vi "Build.vi"(8 "error in (no error)":errorcluster, 11 "Build in":refnum<class "AB_PackedLibrary.lvclass">) -> (0 "error out":errorcluster, 1 "GeneratedFiles":path[](array[path]), 2 "GeneratedDirectories":path[](array[path]), 3 "Build out":refnum<class "AB_PackedLibrary.lvclass">, 4 "GeneratedFileGUIDs":string[](array[string]), 5 "OutputDirectory":path, 7 "Dependencies":T1[](array[typedef]))   [LabVIEW 2020, in "AB_PackedLibrary.lvclass"]
uses:
  <vilib>/AppBuilder/AB_Classes/PackedLib/AB_PackedLibrary.lvclass
  e:/builds/penguin/labview/branches/2020/dev/dist/vi.lib/AppBuilder/AB_Classes/Build/AB_Build.lvclass
  e:/builds/penguin/labview/branches/2020/dev/dist/vi.lib/AppBuilder/AB_Classes/TargetFile/AB_Targetfile.lvclass
  <vilib>/AppBuilder/AB_Dependency.ctl
  <vilib>/Utility/lvfile.llb/LVFileType.ctl
  <vilib>/AppBuilder/AB_Classes/PackedLib/AB_PackedLibrary.lvclass/AB_PackedLibrary.ctl
  <resource>/Framework/Providers/Common/provcom_StringGlobals.vi
  <vilib>/AppBuilder/AB_Classes/Source/AB_Source.lvclass
  <vilib>/AppBuilder/AB_Classes/TargetFile/AB_Targetfile.lvclass
  <vilib>/AppBuilder/AB_Classes/Destination/AB_Destination.lvclass
  <vilib>/AppBuilder/AB_Classes/Build/AB_Build.lvclass
  <vilib>/Utility/lvfile.llb/NI_FileType.lvlib
panel:
  out "error out 2":errorcluster
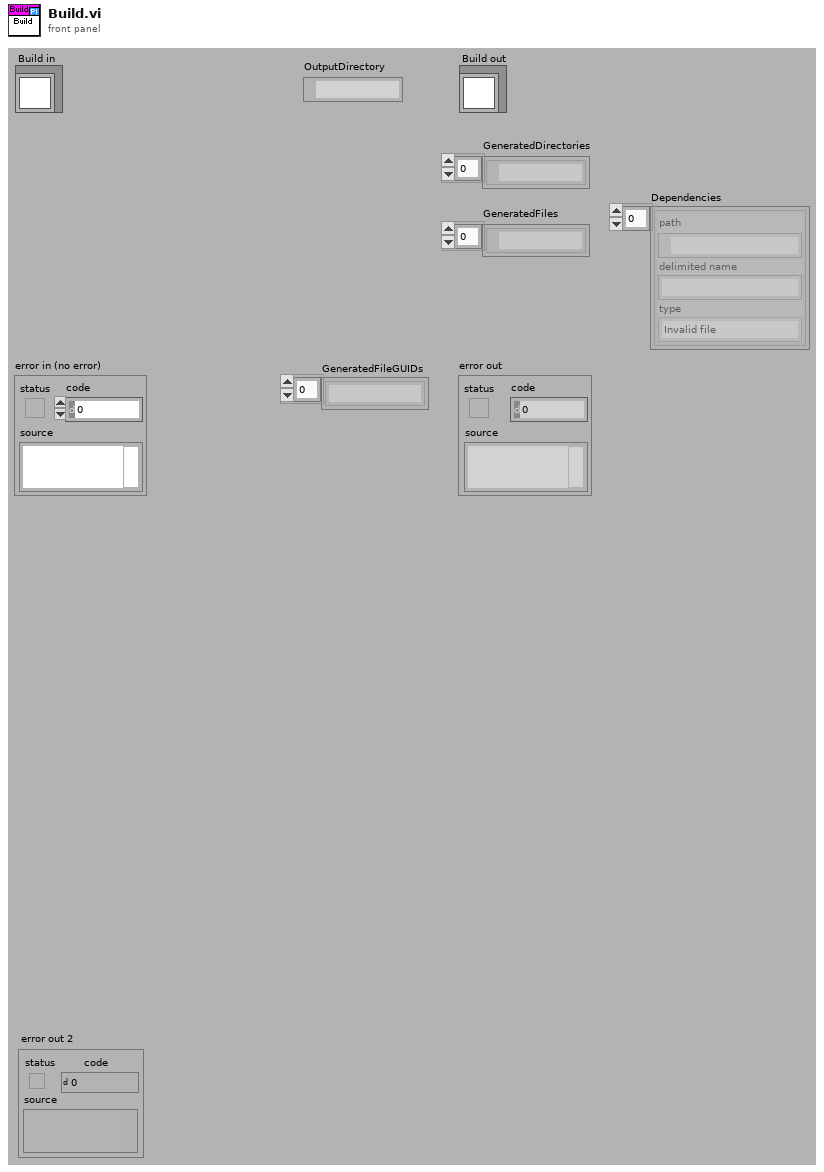
[diagram p1: front panel]
types:
  T1 = typedef "AB_Dependency.ctl" = cluster{"path":path, "delimited name":string, "type":T2}
  T2 = typedef "NI_FileType.lvlib/LVFileType.ctl" = enum32{"Invalid file", "Unknown type", "Instrument", "Control", "Polymorphic VI", "Project", "Library", "LVClass", "XControl", "XNode", "Shared library", ".NET assembly", "ActiveX interface", "CIN", "Run-time menu", "Palette menu", "Help file", "LLB", "XNode Edit Dependency", "Class Private Data Control", "Statechart", "MathScript .m file", "Ladder Diagram", "LVLibp", "XNode Build Dependency"}
  T3 = typedef "AB_Source.ctl" = cluster{"path":path, "itemID":string, "parentIndex":i32, "sourceInclusion":T4, "destinationIndex":i32, "properties":T5[], "newName":string, "lvfile":bool, "valid":bool, "eng_inBuild":bool, "eng_isNonVILink":bool, "Amalgamation":bool, "Amalgamation Piece":bool, "eng_delimitedName":string, "preventRename":bool}
  T4 = typedef "AB_Source_Inclusion.ctl" = enum16{"IncludeIfReferenced", "Include", "Exclude", "TopLevel"}
  T5 = typedef "AB_Source_Properties.ctl" = cluster{"sourcePropertyType":T6, "value":variant}
  T6 = typedef "AB_Source_Property_Type.ctl" = enum16{"Remove block diagram", "Remove front panel", "Password", "Window has title bar", "Show menu bar", "Show vertical scroll bar", "Show horizontal scroll bar", "Show toolbar", "Show Abort button", "Show fp when called", "Window behavior", "Allow user to close window", "Window run-time position", "Run when opened", "Allow debugging", "Auto error handling", "Generate guard code", "Use stack variables", "Expression folding", "Integer only", "Inline subVI"}
  T7 = typedef "AB_Build.ctl" = cluster{"buildSpecName":string, "buildSpecDescription":string, "destinations":refnum<class "AB_Destination.lvclass">[], "exclusionOption":T8, "defaultLanguage":string, "supportedLanguages":string[], "excludedDirectories":path[], "buildContext":refnum<vi>, "buildObject":T9, "preview":bool, "programatic":bool, "progressBarEvents":T10, "userLog_Path":path, "preActionID":string, "preAction_Path":path, "postActionID":string, "postAction_Path":path, "eng_checkForBrokenVIs?":bool, "eng_verboseLinkerErrors?":bool, "localDest_Path":path, "targetDest_Path":path, "removeVIObject":u16, "cache":refnum<class "PreviewCache.lvclass">, "use cache":bool, "previewCache_ID":string, "buildCache_ID":string, "eng_TempLocalDest_Path":path, "eng_collectDependencies?":bool, "versionInfo":cluster{"buildVersion":cluster{"major":u16, "minor":u16, "patch":u16, "build":u16}, "autoIncrement":bool}, "eng_enableVIChecksums":bool}
  T8 = typedef "AB_Exclusion_Option.ctl" = cluster{"typedefs":bool, "polymorphicVIs":bool, "unusedLibraryItems":bool, "modifyLibraryFile":bool, "edit-timeDependencies":bool, "inlineVIs":bool, "dependent PPLs":bool, "dependent DLLs":bool}
  T9 = typedef "ItemRef.ctl" = u64
  T10 = typedef "provcom_ProgressBar_Events.ctl" = cluster{"newJob":refnum<user-event>, "newItem":refnum<user-event>, "errorMsg":T11, "cancel":refnum<user-event>}
  T11 = typedef "mxLvBuildError.ctl" = refnum<user-event>
  T12 = typedef "AB_Targetfile.ctl" = cluster{"targetfileName":string, "targetfileGUID":string, "enableDebugging":bool, "versionInfo":cluster{"productName":string, "legalCopyright":string, "companyName":string, "internalName":string, "fileDescription":string}, "eng_consolidatedTypeInfo":string, "fastFileFormat":bool, "eng_LEIFBuildData":u32, "versionIndependent":bool}
  T13 = typedef "AB_CopyFiles_Data.ctl" = cluster{"processedItems":T14[]}
  T14 = typedef "AB_Source_Processed_Info.ctl" = cluster{"destPath":path, "buildDelimitedName":string, "sourceIndex":i32, "topLevel":bool}
  T15 = typedef "AB_Destination.ctl" = cluster{"destName":string, "path":path, "libraryName":string, "preserveHierarchy":bool, "eng_inBuild":bool, "eng_libraryReference":refnum<vi>, "eng_restictAddToNewLibrary":bool}
  T16 = typedef "AB_Version_Info.ctl" = cluster{"PrivateBuild":string, "SpecialBuild":string, "LegalCopyright":string, "LegalTrademarks":string, "Comments":string, "FileDescription":string, "InternalName":string, "file version":cluster{"major":u16, "minor":u16, "patch":u16, "build":u16}, "ProductName":string, "FileType":u16, "CompanyName":string, "OriginalFilename":string}
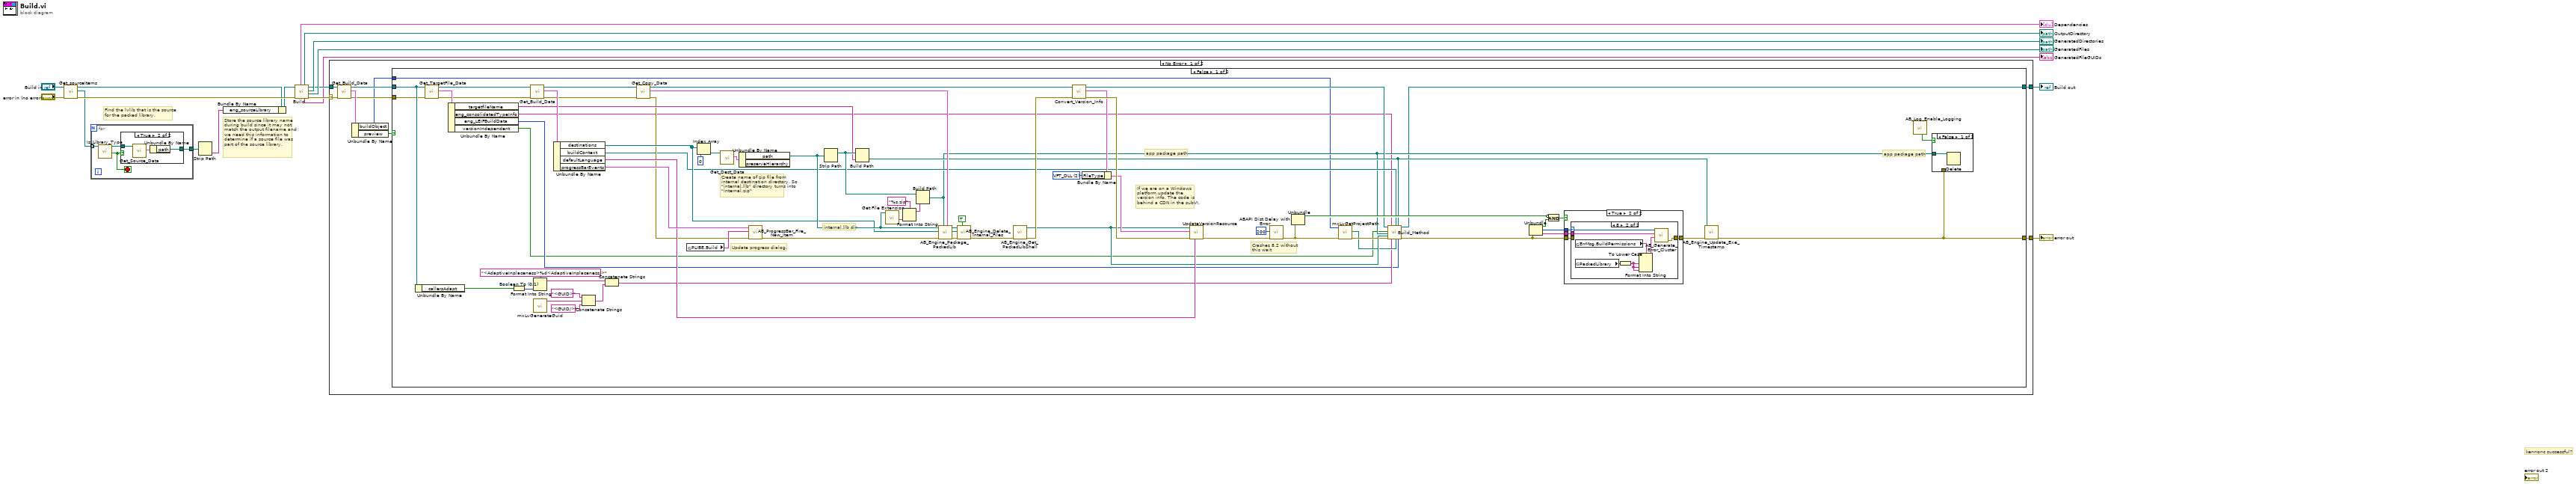
[diagram p0: block diagram]
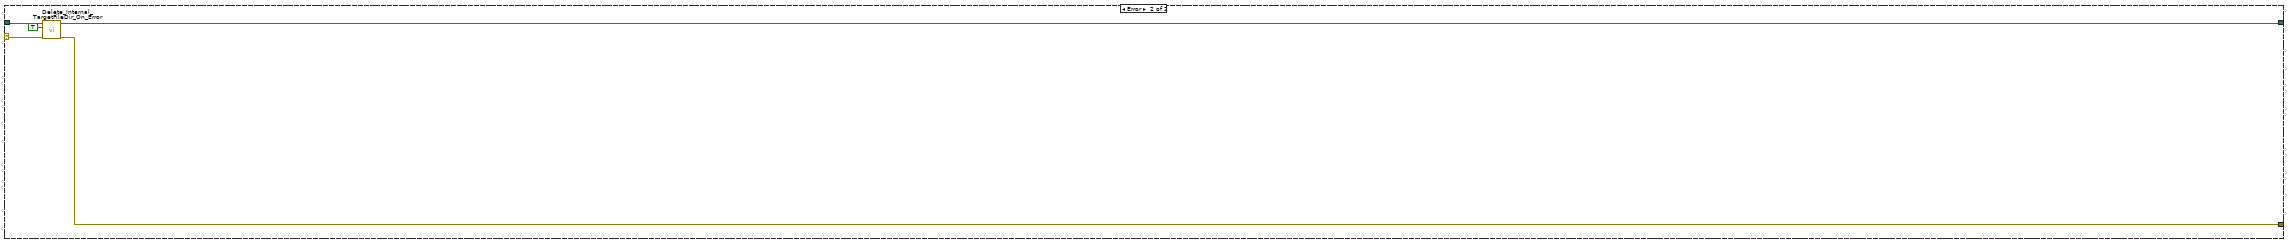
[diagram p7: hidden frame]
diagram:
  # "Store the source library name during build since it may not match the output filename and we need this information to determine if a source file was part of the source library."
  # "Find the lvlib that is the source for the packed library."
  # "kennonc successful?"
  n1 = call <vilib>:"Get_sourceItems.vi"("error in (no error)"="error in (no error)", "Class in"="Build in") -> ("error out"=w7:errorcluster, "sourceItems"=w6:refnum<class "AB_Source.lvclass">[], "Class out"=w4:refnum<class "AB_PackedLibrary.lvclass">)  [unwired: 7 in]
  n2 = for {
    tunnel: w6 -> [w21] mode=indexing
    tunnel: [w19] -> w5
    stop <- w18 stop-if-true
    n3 = call-dynamic "Is_Library_Type.vi"("AB_Source in"=w21) -> ("LVLIBPtopLevel"=w18:bool, "AB_Source out"=w20:refnum<class "AB_Source.lvclass">)  [unwired: 1 in, 8 out]
    n4 = case shown="True" w18 {
      tunnel: w20 -> [_ w22]
      tunnel: [_ w24] -> w19
      frame False {
      }
      frame True {
        n5 = call <vilib>:"Get_Source_Data.vi"("Class in"=w22) -> ("data"=w23:T3)  [unwired: 1 in, 9 out]
        n6 = Unbundle By Name(w23) -> ("path"=w24:path)
      }
    }
  }
  n7 = Strip Path(path=w5) -> (name=w2:string)  [unwired: 1 out]
  n8 = Bundle By Name(cluster=w4, "eng_sourceLibrary"=w2) -> (w3:refnum<class "AB_PackedLibrary.lvclass">)
  n9 = call-parent "Build.vi"("error in (no error)"=w7, "Build in"=w3) -> ("error out"=w12:errorcluster, "GeneratedFiles"=→"GeneratedFiles":path[], "GeneratedDirectories"=→"GeneratedDirectories":path[], "Build out"=w13:refnum<class "AB_PackedLibrary.lvclass">, "GeneratedFileGUIDs"=→"GeneratedFileGUIDs":string[], "OutputDirectory"=→"OutputDirectory":path, "Dependencies"=→"Dependencies":T1[])  [unwired: 3 out]
  n10 = case shown="No Error" w12 {
    selector: w12 -> [w27 w121]
    tunnel: [w33 w119] -> w15
    tunnel: [w32 w120] -> w14
    tunnel: w13 -> [w31 w122]
    frame No Error {
      n11 = call <vilib>:"Get_Build_Data.vi"("error in (no error)"=w27, "Class in"=w31) -> ("error out"=w26:errorcluster, "data"=w30:T7, "Class out"=w28:refnum<class "AB_PackedLibrary.lvclass">)  [unwired: 7 out]
      n12 = Unbundle By Name(w30) -> ("buildObject"=w25:T9, "preview"=w29:bool)
      n13 = case shown="False" w29 {
        tunnel: [w37 w117] -> w33
        tunnel: [w38 w116] -> w32
        tunnel: w28 -> [w83 w117]
        tunnel: w26 -> [w82 w116]
        tunnel: w25 -> [w46 _]
        frame False {
          w97 = u16 2 items=["VFT_UNKNOWN", "VFT_APP", "VFT_DLL", "VFT_DRV", "VFT_FONT", "VFT_VXD", "-", "VFT_STATIC_LIB"] ("FileType")
          # "app package path"
          # "Crashes 8.2 without\nthis wait"
          # "Create name of zip file from internal destination directory. So \"internal.llb\" directory turns into \"internal.zip\""
          # "internal.llb dir"
          # "app package path"
          # "Update progress dialog."
          # "If we are on a Windows platform,update the version info. The code is behind a CDN in the subVI."
          n14 = Unbundle By Name(w83) -> ("callersAdapt"=w57:bool)
          n15 = call <vilib>:"Get_TargetFile_Data.vi"("error in (no error)"=w82, "AB_Targetfile in"=w83) -> ("error out"=w81:errorcluster, "data"=w84:T12, "AB_Targetfile out"=w79:refnum<class "AB_PackedLibrary.lvclass">)  [unwired: 7 in]
          n16 = Unbundle By Name(w84) -> ("targetfileName"=w80:string, "eng_consolidatedTypeInfo"=w49:string, "eng_LEIFBuildData"=w35:u32, "versionIndependent"=w34:bool)
          n17 = Boolean To (0,1)(Boolean=w57) -> (0, 1=w56:i16)
          n18 = call <vilib>:"Get_Build_Data.vi"("error in (no error)"=w81, "Class in"=w79) -> ("error out"=w62:errorcluster, "data"=w99:T7, "Class out"=w64:refnum<class "AB_PackedLibrary.lvclass">)  [unwired: 7 out]
          n19 = Format Into String(format string="<AdaptiveInplaceness>%d<AdaptiveInplaceness/>", w56) -> (resulting string=w44:string)  [unwired: 2 in, 1 out]
          n20 = call <resource>:"mxLvGenerateGuid.vi"() -> ("Value"=w42:string)  [unwired: 10 in, 1 out]
          n21 = Unbundle By Name(w99) -> ("destinations"=w85:refnum<class "AB_Destination.lvclass">[], "buildContext"=w54:refnum<vi>, "defaultLanguage"=w86:string, "progressBarEvents"=w94:T10)
          n22 = Concatenate Strings("<GUID>" ("string"), w42, "<GUID/>" ("string")) -> (w39:string)
          n23 = Concatenate Strings(w44, w39) -> (w43:string)
          n24 = call <vilib>:"Get_Copy_Data.vi"("error in (no error)"=w62, "AB_Build in"=w64) -> ("error out"=w61:errorcluster, "copyData"=w60:T13, "AB_Build out"=w63:refnum<class "AB_PackedLibrary.lvclass">)  [unwired: 7 in]
          n25 = global read "provcom_StringGlobals.vi" "PLIBE.Build"() -> (w95:string)
          n26 = Index Array(array=w85, index=0) -> (element=w89:refnum<class "AB_Destination.lvclass">)
          n27 = call <vilib>:"Get_Dest_Data.vi"("Class in"=w89) -> ("destName"=w100:T15)  [unwired: 1 in, 9 out]
          n28 = Unbundle By Name(w100) -> ("path"=w88:path)  [unwired: 1 out]
          n29 = call <vilib>:"AB_ProgressBar_Fire_New_Item.vi"("error in (no error)"=w61, "Label"=w95, "progressBarEvents in"=w94) -> ("error out"=w92:errorcluster)  [unwired: 8 out]
          n30 = Strip Path(path=w88) -> (stripped path=w90:path)  [unwired: 1 out]
          n31 = Build Path(base path=w90, name or relative path=w80) -> (appended path=w55:path)
          n32 = call <vilib>:"Get File Extension.vi"("file"=w88) -> ("filename without extension"=w70:string)  [unwired: 1 in, 9 out]
          n33 = Format Into String(format string="%s.zip", w70) -> (resulting string=w69:string)  [unwired: 2 in, 1 out]
          n34 = Build Path(base path=w90, name or relative path=w69) -> (appended path=w52:path)
          n35 = call <vilib>:"AB_Engine_Package_PackedLib.vi"("processed_sourceItems"=w60, "application package path"=w52, "error in (no error)"=w92, "destinations"=w85, "internal directory"=w88) -> ("error out"=w67:errorcluster, "support dir"=w65:path, "dup internal directory"=w66:path)  [unwired: 4 in]
          n36 = call <vilib>:"AB_Engine_Delete_Internal_Files.vi"("override Mac support directory preservation"=TRUE ("is Packed Library?"), "error in (no error)"=w67, "support dir"=w65, "internal directory"=w66) -> ("error out"=w91:errorcluster)  [unwired: 7 in]
          n37 = call <vilib>:"AB_Engine_Get_PackedLibShell.vi"("error in (no error)"=w91) -> ("error out"=w78:errorcluster, "pathPackedLibShell"=w51:path)  [unwired: 9 in]
          n38 = call-dynamic "Convert_Version_Info.vi"("error in (no error)"=w78, "AB_Targetfile in"=w63) -> ("error out"=w98:errorcluster, "input version info"=w96:T16, "AB_Targetfile out"=w53:refnum<class "AB_PackedLibrary.lvclass">)  [unwired: 7 out]
          n39 = Bundle By Name(cluster=w96, "FileType"=w97) -> (w93:T16)
          n40 = call <resource>:"UpdateVersionResource.vi"("default language"=w86, "error in (no error)"=w98, "input version info"=w93, "path"=w51) -> ("error out"=w87:errorcluster)  [unwired: 1 in, 6 out]
          n41 = call <vilib>:"ABAPI Dist Delay with Error.vi"("error in (no error)"=w87, "milliseconds to wait"=u32 200) -> ("error out"=w48:errorcluster)  [unwired: 1 in, 8 out]
          n42 = Unbundle(w48) -> ("status"=w75:bool)  [unwired: 2 out]
          n43 = call <resource>:"mxLvGetProjectPath.vi"("error in"=w48, "Item"=w46) -> ("error out"=w47:errorcluster, "Project Path"=w45:path)  [unwired: 7 in, 1 out]
          n44 = call-dynamic "Build_Method.vi"("AB_PackedLibrary in"=w53, "versionIndependent"=w34, "Zip path"=w52, "Shell Path"=w51, "error in (no error)"=w47, "eng_consolidatedTypeInfo"=w49, "Options string"=w43, "buildContext"=w54, "source project path"=w45, "PackedLib path"=w55, "eng_LEIFBuildDataCookie"=w35) -> ("AB_PackedLibrary out"=w37:refnum<class "AB_PackedLibrary.lvclass">, "error out"=w50:errorcluster)  [unwired: 7 in]
          n45 = Unbundle(w50) -> ("status"=w74:bool, "code"=w72:i32, "source"=w71:string)
          n46 = Compound Arithmetic op=AND(invert w75, w74) -> (w73:bool)
          n47 = case shown="True" w73 {
            tunnel: w50 -> [w103 w106]
            tunnel: w72 -> [_ w107]
            tunnel: [w103 w105] -> w77
            tunnel: w71 -> [_ w104]
            frame False {
            }
            frame True {
              n48 = case shown="8" w107 {
                selector: w107 -> [_ w115]
                tunnel: w106 -> [w108 _]
                tunnel: [w108 w113] -> w105
                tunnel: w104 -> [_ w114]
                frame Default {
                }
                frame 8 {
                  n49 = global read "provcom_StringGlobals.vi" "ErrMsg.BuildPermissions"() -> (w111:string)
                  n50 = global read "provcom_StringGlobals.vi" "PackedLibrary"() -> (w110:string)
                  n51 = To Lower Case(string=w110) -> (all lower case string=w112:string)
                  n52 = Format Into String(format string=w111, w112, w112, w112) -> (resulting string=w109:string)  [unwired: 2 in, 1 out]
                  n53 = call <vilib>:"AB_Generate_Error_Cluster.vi"("Additional Message"=w109, "source"=w114, "Code"=w115) -> ("error out"=w113:errorcluster)  [unwired: 1 in, 7 out]
                }
              }
            }
          }
          n54 = call <vilib>:"AB_Engine_Update_Exe_Timestamp.vi"("error in (no error)"=w77, "pathExe"=w55) -> ("error out"=w38:errorcluster)  [unwired: 9 out]
          n55 = call <vilib>:"AB_Log_Enable_Logging.vi"() -> ("keep internal.llb"=w59:bool)  [unwired: 2 in, 9 out]
          n56 = case shown="False" w59 {
            tunnel: w38 -> [_ _]
            tunnel: w52 -> [w102 _]
            frame False {
              n57 = Delete(path (use dialog)=w102) -> ()  [unwired: 4 in, 3 out]
            }
            frame True {
            }
          }
        }
        frame True {
        }
      }
    }
    frame Error {
      n58 = call-dynamic "Delete_Internal_TargetFileDir_On_Error.vi"("error in (no error)"=w121, "override Mac support directory preservation"=TRUE ("delete Mac support directory"), "Build in"=w122) -> ("error out"=w120:errorcluster, "Build out"=w119:refnum<class "AB_PackedLibrary.lvclass">)  [unwired: 7 in]
    }
  }
  "error out" <- w14
  "Build out" <- w15
